vi "ZCAN_Setfilter.vi"(6 "filter_start":string="0x00000001", 7 "frame_type":T1=enum."Extended frame", 8 "error in (no error)":errorcluster, 9 "filter_end":string="0x1FFFF", 10 "can_index":u32, 11 "device_handle":u32) -> (0 "error out":errorcluster, 3 "SetfilterResult":bool)   [LabVIEW 2020, in "zlgcan.lvlib"]
uses:
  zlgcan.lvlib
  data_type/frame type.ctl
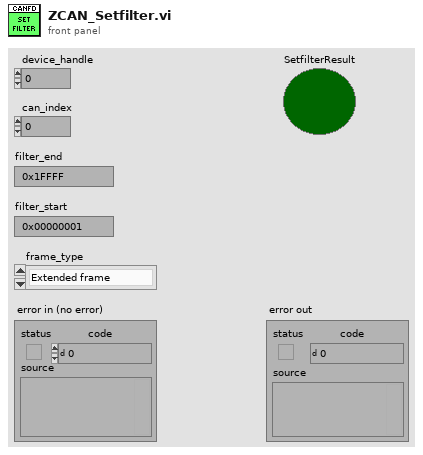
[diagram p1: front panel]
types:
  T1 = typedef "zlgcan.lvlib/frame type.ctl" = enum32{"Standard frame", "Extended frame"}
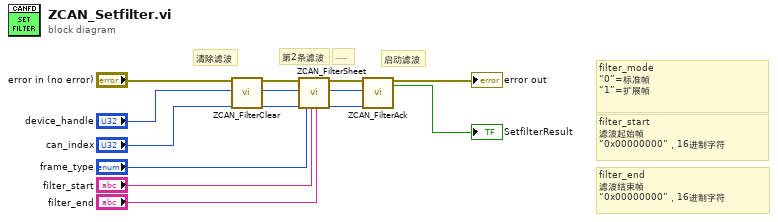
[diagram p0: block diagram]
diagram:
  # "......"
  # "启动滤波"
  # "第2条滤波"
  # "清除滤波"
  # "filter_end\n滤波结束帧\n“0x00000000”，16进制字符"
  # "filter_start   \n滤波起始帧 \n“0x00000000”，16进制字符"
  # "filter_mode\n“0”=标准帧\n“1”=扩展帧"
  n1 = call "ZCAN_FilterClear.vi"("error in (no error)"="error in (no error)", "can_index_handle"="device_handle", "can_index"="can_index") -> ("error out"=w10:errorcluster, "can_index_handle(out)"=w12:u32, "can_index(out)"=w11:u32)  [unwired: 14 in]
  n2 = call "ZCAN_FilterSheet.vi"("error in (no error)"=w10, "can_index_handle"=w12, "can_index"=w11, "filter_mode"="frame_type", "filter_start"="filter_start", "filter_end"="filter_end") -> ("error out"=w6:errorcluster, "can_index_handle（out）"=w5:u32, "can_index (out)"=w4:u32)  [unwired: 11 in]
  n3 = call "ZCAN_FilterAck.vi"("error in (no error)"=w6, "can_index_handle"=w5, "can_index"=w4) -> ("error out"=→"error out":errorcluster, "启动滤波成功？"=→"SetfilterResult":bool)  [unwired: 13 in, 2 out]
